vi "Modem Status Interpret Data.vi"() -> (1 "Subsea Bar Graph":T1 {"Gain" format="%#.0f"; "Signal Quality" format="%#.0f"}, 2 "Topside Bar Graph":T1 {"Gain" format="%#.0f"; "Signal Quality" format="%#.0f"})   [LabVIEW 2011]
uses:
  GUI/Controls/Signal Bar Graph.ctl
  Variable List Modem Status Analog.ctl
panel:
  # "G"
  # "G"
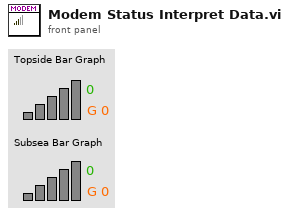
[diagram p1: front panel]
types:
  T1 = typedef "Signal Bar Graph.ctl" = cluster{"Bar Graph":cluster{"Boolean":bool, "Boolean 2":bool, "Boolean 3":bool, "Boolean 4":bool, "Boolean 5":bool}, "Signal Quality":dbl, "Gain":dbl}
  T2 = typedef "Variable List Modem Status Analog.ctl" = enum16{"TS_Signal_Quality", "TS_PCB_Temp", "TS_Gain", "DH_Signal_Quality", "DH_PCB_Temp", "DH_Gain", "Link_Status"}
  T3 = cluster{"[0]":bool, "[1]":bool, "[2]":bool, "[3]":bool, "[4]":bool}
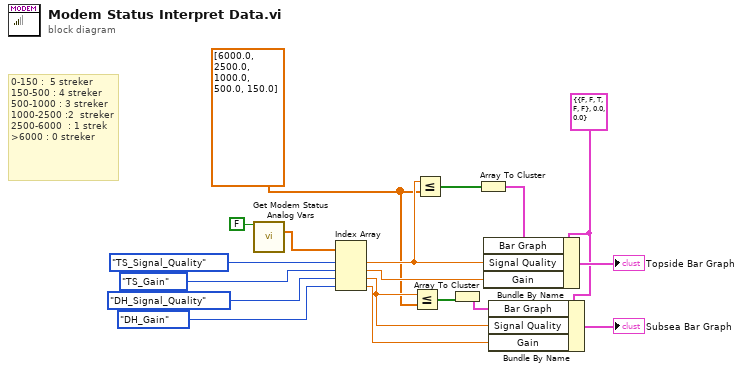
[diagram p0: block diagram]
diagram:
  w3 = dbl[] [6000.0, 2500.0, 1000.0, 500.0, 150.0]
  w10 = T1 {"Bar Graph"={"Boolean"=FALSE, "Boolean 2"=FALSE, "Boolean 3"=TRUE, "Boolean 4"=FALSE, "Boolean 5"=FALSE}, "Signal Quality"=0.0, "Gain"=0.0} ("Bar Graph")
  # "0-150 :  5 streker\n150-500 : 4 streker\n500-1000 : 3 streker\n1000-2500 :2  streker\n2500-6000  : 1 strek\n>6000 : 0 streker"
  n1 = call "Get Modem Status Analog Vars.vi"("Common alarm handling(F)"=FALSE) -> ("Values"=w17:dbl[])  [unwired: 8 in, 6 out]
  n2 = Index Array(array=w17, index #1=Variable_List_Modem_Status_Analog."TS_Signal_Quality" ("Variable ID"), index #2=Variable_List_Modem_Status_Analog."TS_Gain" ("Variable ID"), index #3=Variable_List_Modem_Status_Analog."DH_Signal_Quality" ("Variable ID"), index #4=Variable_List_Modem_Status_Analog."DH_Gain" ("Variable ID")) -> (element #1=w7:dbl, element #2=w16:dbl, element #3=w4:dbl, element #4=w8:dbl)
  n3 = Less Or Equal?(x=w4, y=w3) -> (x <= y?=w2:bool[])
  n4 = Less Or Equal?(x=w7, y=w3) -> (x <= y?=w6:bool[])
  n5 = Array To Cluster(array=w2) -> (cluster=w1:T3)
  n6 = Array To Cluster(array=w6) -> (cluster=w5:T3)
  n7 = Bundle By Name(cluster=w10, "Bar Graph"=w5, "Signal Quality"=w7, "Gain"=w16) -> (→"Topside Bar Graph":T1)
  n8 = Bundle By Name(cluster=w10, "Bar Graph"=w1, "Signal Quality"=w4, "Gain"=w8) -> (→"Subsea Bar Graph":T1)
